vi "Physics Calculator.vi"() -> ()   [LabVIEW 2015]
panel:
  in  "Time":dbl
  out "X Final":dbl
  in  "Acceleration":dbl
  in  "Velocity Inititial":dbl
  in  "X initial":dbl
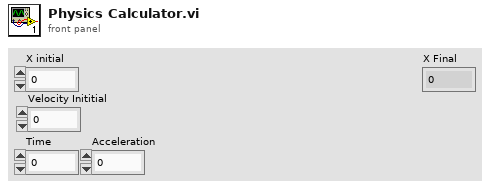
[diagram p1: front panel]
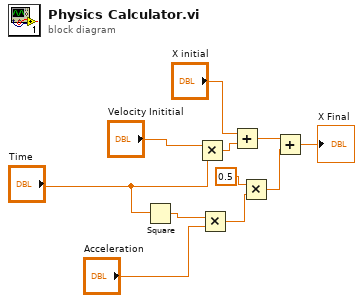
[diagram p0: block diagram]
diagram:
  n1 = Square(x="Time") -> (x^2=w9:dbl)
  n2 = Multiply(x="Velocity Inititial", y="Time") -> (x*y=w2:dbl)
  n3 = Multiply(x=w9, y="Acceleration") -> (x*y=w7:dbl)
  n4 = Add(x="X initial", y=w2) -> (x+y=w4:dbl)
  n5 = Multiply(x=0.5, y=w7) -> (x*y=w5:dbl)
  n6 = Add(x=w4, y=w5) -> (x+y=→"X Final":dbl)
